vi "BuildGraph.vi"(8 "error in (no error)":errorcluster, 9 "pass?":bool, 10 "reference":refnum<class "Game.lvclass">, 11 "object in":refnum<class "Utilities.lvclass">) -> (0 "error out":errorcluster, 2 "Intensity Graph":dbl[][](graph), 3 "object out":refnum<class "Utilities.lvclass">)   [LabVIEW 2023, in "Utilities.lvclass"]
uses:
  Utilities.lvclass
  Game_class/Game.lvclass
  Game_class/Game.lvclass/Game.ctl
  Game_class/Read FieldRef.vi
  Field_class/Field.lvclass
panel:
  in  "Threshold":i32=200
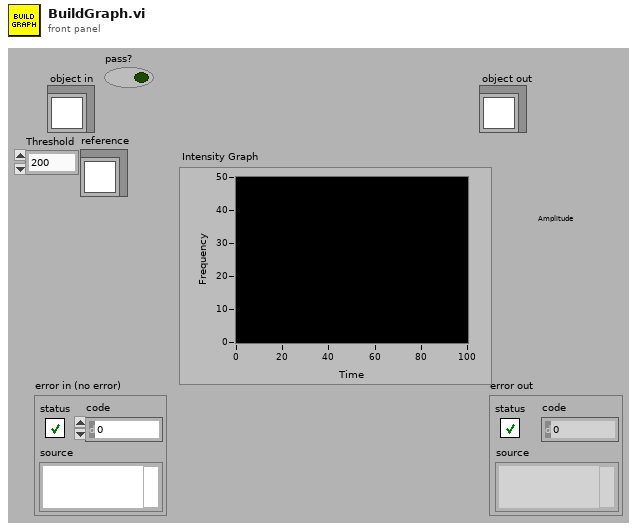
[diagram p1: front panel]
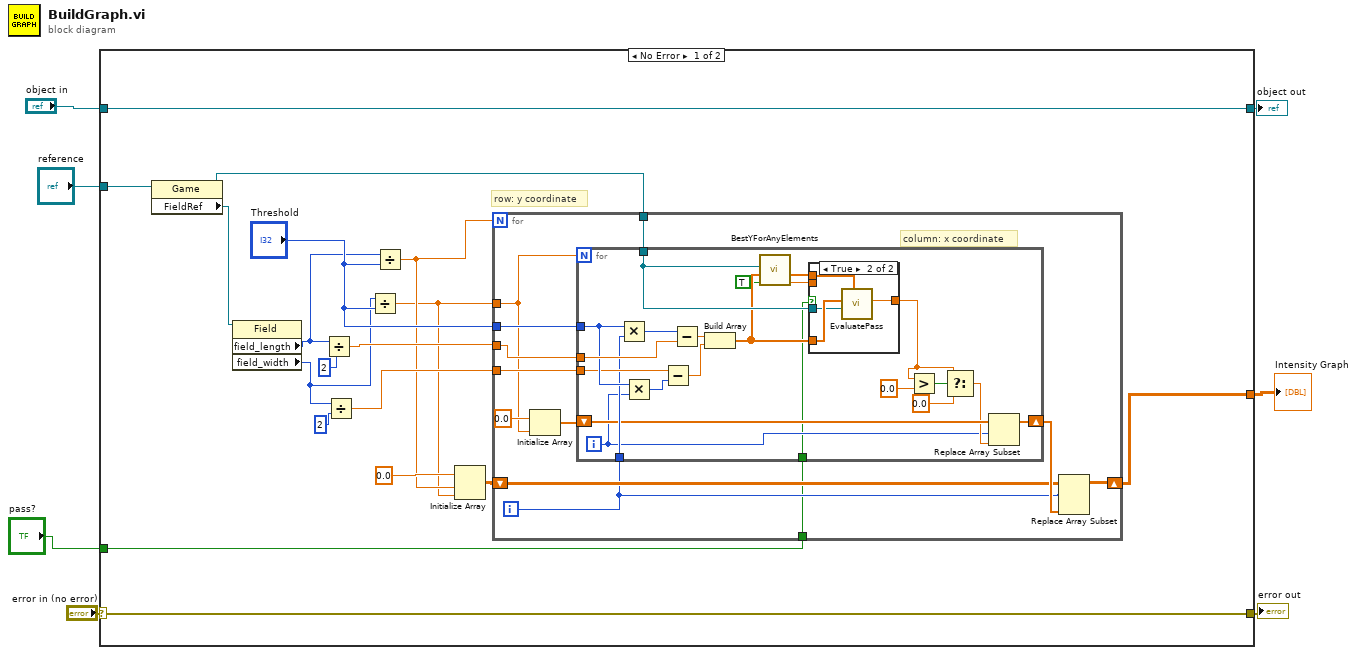
[diagram p0: block diagram]
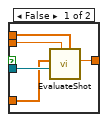
[diagram p2: hidden frame]
diagram:
  n1 = case shown="No Error" "error in (no error)" {
    selector: "error in (no error)" -> [w25 w70]
    tunnel: [w25 w70] -> w6
    tunnel: [w24 w69] -> w4
    tunnel: "object in" -> [w24 w69]
    tunnel: [w11 _] -> w3
    tunnel: "reference" -> [w10 _]
    tunnel: "pass?" -> [w8 _]
    frame No Error {
      # "row: y coordinate"
      n2 = property class="Game"(reference=w10) -> (reference out=w9:refnum<class "Game.lvclass">, "FieldRef"=w23:refnum<class "Field.lvclass">)  [unwired: 1 in, 1 out]
      n3 = property class="Field"(reference=w23) -> ("field_length"=w16:i32, "field_width"=w19:i32)  [unwired: 1 in, 2 out]
      n4 = Divide(x=w16, y=2) -> (x/y=w20:dbl)
      n5 = Divide(x=w19, y=2) -> (x/y=w17:dbl)
      n6 = Divide(x=w19, y="Threshold") -> (x/y=w12:dbl)
      n7 = Divide(x=w16, y="Threshold") -> (x/y=w13:dbl)
      n8 = Initialize Array(0.0 ("element"), w13, w12) -> (w14:dbl[][])
      n9 = for {
        N: w13 -> [_]
        shift-right: [w27] -> w11
        shift-left: w14 -> [w29]
        tunnel: "Threshold" -> [w37]
        tunnel: w20 -> [w36]
        tunnel: w17 -> [w35]
        tunnel: w12 -> [w32]
        tunnel: w9 -> [w34]
        tunnel: w8 -> [w26]
        i -> [w28]
        # "column: x coordinate"
        n10 = Initialize Array(0.0 ("element"), w32) -> (w31:dbl[])
        n11 = for {
          N: w32 -> [_]
          shift-right: [w45] -> w30
          shift-left: w31 -> [w48]
          tunnel: w37 -> [w57]
          tunnel: w36 -> [w58]
          tunnel: w35 -> [w56]
          tunnel: w28 -> [w52]
          tunnel: w34 -> [w43]
          tunnel: w26 -> [w38]
          i -> [w46]
          n12 = Multiply(x=w57, y=w52) -> (x*y=w59:i32)
          n13 = Multiply(x=w57, y=w46) -> (x*y=w55:i32)
          n14 = Subtract(x=w56, y=w55) -> (x-y=w53:dbl)
          n15 = Subtract(x=w59, y=w58) -> (x-y=w54:dbl)
          n16 = Build Array(w54, w53) -> (w42:dbl[])
          n17 = call "BestYForAnyElements.vi"("inimigos"=TRUE, "Position to be analyzed"=w42, "Game"=w43) -> ("Best y"=w41:dbl, "Gap Coord"=w40:dbl[])  [unwired: 5 in, 2 out]
          n18 = case shown="True" w38 {
            tunnel: [w64 w65] -> w44
            tunnel: w43 -> [w63 w66]
            tunnel: w42 -> [w62 w67]
            tunnel: w41 -> [w61 _]
            tunnel: w40 -> [w60 w68]
            frame False {
              n19 = call "EvaluateShot.vi"("Gap Coord"=w60, "BestY"=w61, "Game"=w63, "Point"=w62) -> ("Evaluation"=w64:dbl)  [unwired: 5 in, 2 out]
            }
            frame True {
              n20 = call "EvaluatePass.vi"("Gap Coord"=w68, "Game"=w66, "Point"=w67) -> ("evaluation"=w65:dbl)  [unwired: 6 in, 2 out]
            }
          }
          n21 = Greater?(x=w44, y=0.0) -> (0:w51:bool)
          n22 = Select(t=w44, s=w51, f=0.0) -> (s? t:f=w47:dbl)
          n23 = Replace Array Subset(array=w48, new element=w47, index=w46) -> (w45:dbl[])
        }
        n24 = Replace Array Subset(array=w29, new element=w30, index (row)=w28) -> (w27:dbl[][])  [unwired: 1 in]
      }
    }
    frame Error {
    }
  }
  "error out" <- w6
  "object out" <- w4
  "Intensity Graph" <- w3
